vi "Finalize Spawn.vi"(8 "Error in":errorcluster, 10 "Attributes":refnum<data-value>, 11 "TEMPLATE Actor in":refnum<class "TEMPLATE Actor.lvclass">) -> (0 "Error out":errorcluster, 3 "TEMPLATE Actor out":refnum<class "TEMPLATE Actor.lvclass">)   [LabVIEW 2020, in "_Template.lvlib" / "Templates.lvlib" / "TEMPLATE jettl Actor.lvlib" / "TEMPLATE Actor.lvlib" / "TEMPLATE Actor.lvclass"]
uses:
  TEMPLATE Actor.lvclass
  TEMPLATE Actor.lvclass/TEMPLATE Actor.ctl
  jettl/jettl/jettl.lvlib
  jettl/jettl/Transport/Transport.lvclass
  jettl/jettl/Actor/Actor.lvclass
  jettl/jettl/Actor Attributes.ctl
  jettl/jettl/Msg/Msg.lvclass
  jettl/jettl/Msgs.ctl
  jettl/jettl/Unified Layer.ctl
panel:
  # "This front panel should not be manipulated."
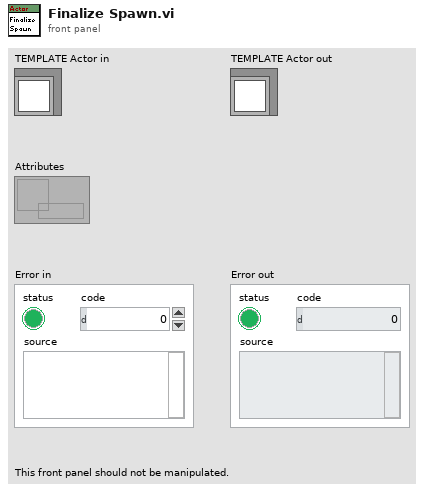
[diagram p1: front panel]
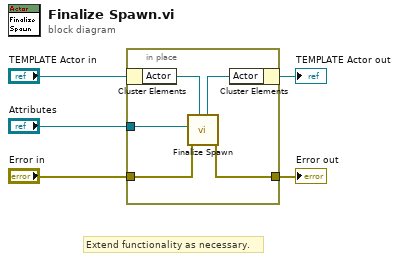
[diagram p0: block diagram]
diagram:
  # "Extend functionality as necessary."
  n1 = in-place {
    in-place-border: "Error in" -> [w7]
    in-place-border: [w6] -> w2
    in-place-border: "Attributes" -> [w8]
    n2 = in-place-cluster #1("TEMPLATE Actor in") -> ("Actor"=w10:refnum<data-value>)
    n3 = call "Finalize Spawn.vi"("Actor in"=w10, "Error in"=w7, "Attributes"=w8) -> ("Error out"=w6:errorcluster, "Actor out"=w9:refnum<data-value>)  [unwired: 7 in]
    n4 = in-place-cluster #1("Actor"=w9) -> (→"TEMPLATE Actor out":refnum<class "TEMPLATE Actor.lvclass">)
  }
  "Error out" <- w2
